vi "Get Audio File Position.vi"(8 "error in (no error)":errorcluster, 11 "Audio File Refnum In":refnum<file>) -> (0 "error out":errorcluster, 2 "Frame Position":u64, 3 "Audio File Refnum Out":refnum<file>)   [LabVIEW 2020, in "G-Audio.lvlib"]
doc: "Get the current read position of the file. The position is in absolute PCM frames (samples/ch).\n\n<b>Note:</b> The read position for Ogg Vorbis files is not sample accurate. Seeking to a position and then reading the position can return a different value."
uses:
  G-Audio.lvlib
  <vilib>/Utility/error.llb/Error Cluster From Error Code.vi
  lib/g_audio_x86.dll
  lib/g_audio_x64.dll
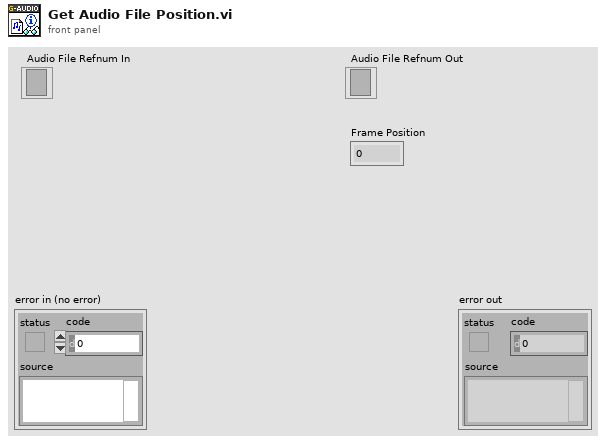
[diagram p1: front panel]
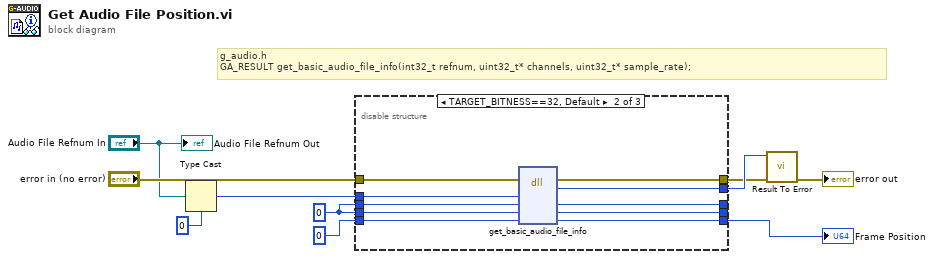
[diagram p0: block diagram]
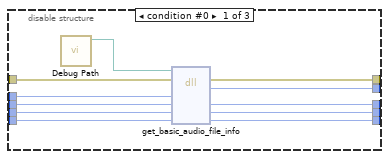
[diagram p2: hidden frame]
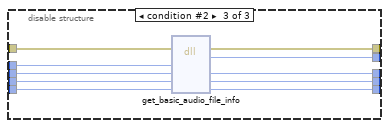
[diagram p3: hidden frame]
diagram:
  w6 = u32 0
  # "g_audio.h\nGA_RESULT get_basic_audio_file_info(int32_t refnum, uint32_t* channels, uint32_t* sample_rate);"
  n1 = Type Cast(type=0, x="Audio File Refnum In") -> (*(type *) &x=w7:i32)
  n2 = disable-structure shown="TARGET_BITNESS==32, Default" {
    disable-tunnel: "error in (no error)" -> [w21 w31 w41]
    disable-tunnel: [w14 w24 w34] -> w5
    disable-tunnel: [w20 w30 w40] -> w4
    disable-tunnel: [w15 w25 w35] -> _
    disable-tunnel: w7 -> [w19 w29 w39]
    disable-tunnel: w6 -> [w18 w28 w38]
    disable-tunnel: w6 -> [w17 w27 w37]
    disable-tunnel: [w16 w26 w36] -> _
    disable-tunnel: u64 0 -> [w12 w23 w33]
    disable-tunnel: [w11 w22 w32] -> w1
    frame condition #0 {
      n3 = call "Debug Path.vi"() -> ("Debug Path"=w13:path)  [unwired: 11 in]
      n4 = dll-call lib="?" fn="get_basic_audio_file_info"(path in=w13, error in=w21, "refnum"=w19, "channels"=w18, "sample_rate"=w17, "read_offset"=w12) -> (error out=w20:errorcluster, "result"=w14:i32, "channels"=w16:u32, "sample_rate"=w15:u32, "read_offset"=w11:u64)  [unwired: 2 in, 1 out]
    }
    frame condition #1 (active) {
      n5 = dll-call lib="C:/github/dataflowg/g-audio/src/LabVIEW/G-Audio/lib/g_audio_x86.*" fn="get_basic_audio_file_info"(error in=w31, "refnum"=w29, "channels"=w28, "sample_rate"=w27, "read_offset"=w23) -> (error out=w30:errorcluster, "result"=w24:i32, "channels"=w26:u32, "sample_rate"=w25:u32, "read_offset"=w22:u64)  [unwired: 3 in, 1 out]
    }
    frame condition #2 {
      n6 = dll-call lib="C:/github/dataflowg/g-audio/src/LabVIEW/G-Audio/lib/g_audio_x64.*" fn="get_basic_audio_file_info"(error in=w41, "refnum"=w39, "channels"=w38, "sample_rate"=w37, "read_offset"=w33) -> (error out=w40:errorcluster, "result"=w34:i32, "channels"=w36:u32, "sample_rate"=w35:u32, "read_offset"=w32:u64)  [unwired: 3 in, 1 out]
    }
  }
  "Frame Position" <- w1
  n7 = call "Result To Error.vi"("error in (no error)"=w4, "Result Code"=w5) -> ("error out"=→"error out":errorcluster)  [unwired: 9 in]
  "Audio File Refnum Out" <- "Audio File Refnum In"
